vi "Gyro Crossover.vi"(1 "Gyro Value":dbl, 2 "Previous Value":dbl) -> (0 "Gyro Value":dbl)   [LabVIEW 2015]
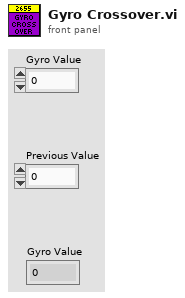
[diagram p1: front panel]
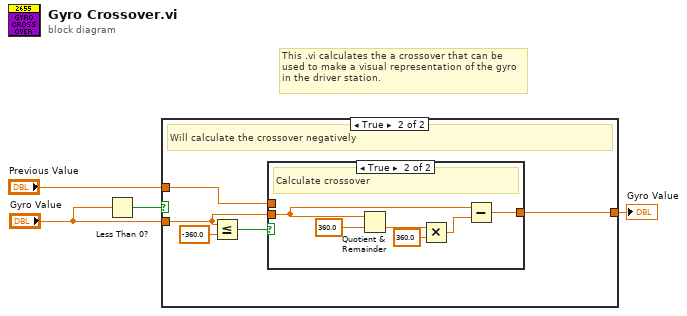
[diagram p0: block diagram]
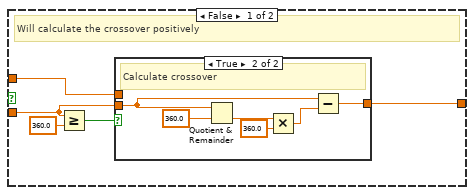
[diagram p2: hidden frame]
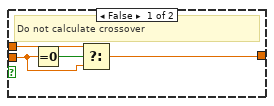
[diagram p3: hidden frame]
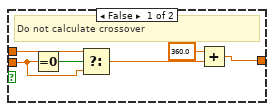
[diagram p4: hidden frame]
diagram:
  # "This .vi calculates the a crossover that can be used to make a visual representation of the gyro in the driver station."
  n1 = Less Than 0?(x="Gyro Value") -> (x < 0?=w2:bool)
  n2 = case shown="True" w2 {
    tunnel: "Previous Value" -> [w7 w21]
    tunnel: "Gyro Value" -> [w6 w22]
    tunnel: [w5 w20] -> w1
    frame False {
      # "Will calculate the crossover positively"
      n3 = Greater Or Equal?(x=w6, y=360.0) -> (x >= y?=w9:bool)
      n4 = case shown="True" w9 {
        tunnel: w6 -> [w11 w16]
        tunnel: [w10 w17] -> w5
        tunnel: w7 -> [w12 _]
        frame False {
          # "Do not calculate crossover"
          n5 = Equal To 0?(x=w11) -> (x = 0?=w13:bool)
          n6 = Select(t=w12, s=w13, f=w11) -> (s? t:f=w10:dbl)
        }
        frame True {
          # "Calculate crossover"
          n7 = Quotient & Remainder(x=w16, y=360.0) -> (floor(x/y)=w14:dbl)  [unwired: 1 out]
          n8 = Multiply(x=w14, y=360.0) -> (x*y=w18:dbl)
          n9 = Subtract(x=w16, y=w18) -> (x-y=w17:dbl)
        }
      }
    }
    frame True {
      # "Will calculate the crossover negatively"
      n10 = Less Or Equal?(x=w22, y=-360.0) -> (x <= y?=w24:bool)
      n11 = case shown="True" w24 {
        tunnel: w22 -> [w28 w33]
        tunnel: [w25 w34] -> w20
        tunnel: w21 -> [w29 _]
        frame False {
          # "Do not calculate crossover"
          n12 = Equal To 0?(x=w28) -> (x = 0?=w30:bool)
          n13 = Select(t=w29, s=w30, f=w28) -> (s? t:f=w26:dbl)
          n14 = Add(x=360.0, y=w26) -> (x+y=w25:dbl)
        }
        frame True {
          # "Calculate crossover"
          n15 = Quotient & Remainder(x=w33, y=360.0) -> (floor(x/y)=w31:dbl)  [unwired: 1 out]
          n16 = Multiply(x=w31, y=360.0) -> (x*y=w35:dbl)
          n17 = Subtract(x=w33, y=w35) -> (x-y=w34:dbl)
        }
      }
    }
  }
  "Gyro Value" <- w1
